vi "PC_SVG DAQ1 to TDVM DAQ2 RSS.vi"() -> ()   [LabVIEW 2021]
uses:
  Synchronization/Typedefs/Routing Path.ctl
  Synchronization/Typedefs/Routing Signal.ctl
  Signal Voltage Generation/Typedefs/Signal Generation Settings.ctl
  Signal Voltage Generation/Typedefs/Generation Types.ctl
  Signal Voltage Generation/Typedefs/Single Tone Settings.ctl
  Signal Voltage Generation/Typedefs/Waveform Type.ctl
  Signal Voltage Generation/Typedefs/Tone Settings.ctl
  Time Domain Measurement/Typedefs/Time Domain Measurements.ctl
  Time Domain Measurement/Typedefs/Timing & Trigger Settings.ctl
  Time Domain Measurement/Typedefs/Timing Settings.ctl
  Time Domain Measurement/Typedefs/Trigger Settings.ctl
  Time Domain Measurement/Typedefs/Execution Settings.ctl
  Common/Typedefs/Execution Options - Measure.ctl
  Time Domain Measurement/Typedefs/Range and Terminal Settings.ctl
  Time Domain Measurement/Typedefs/Specific Channel Settings.ctl
  Time Domain Measurement/DAQ_Time Domain Measurement.lvlib
  Synchronization/DAQ_Synchronization.lvlib
  Signal Voltage Generation/DAQ_Signal Voltage Generation.lvlib
panel:
  in  "Timing and Trigger Settings":T1={"Timing Settings"={"Sample Clock Source"="/Dev2/PFI1", "Sample Rate(Hz)"=100000.0, "Number of Samples"=10000, "Sample Timing Engine"=enum."Auto"}, "Trigger Settings"={"Trigger Type"=enum."Digital Start", "Digital Start Trigger Source"="/Dev2/PFI0", "Digital Start Trigger Edge"=10280}} {"Trigger Settings"."Digital Start Trigger Edge" items=["Rising"=10280, "Falling"=10171]; "Timing Settings"."Sample Rate(Hz)" format="%.2p"}
  out "error out":errorcluster
  out "Time Domain Measurements":T4={"Mean DC Voltage (V)"=[1.0316878948057864], "Vpp Amplitude(V)"=[2.0060539436845626], "Voltage Frequency(Hz)"=[99.99092141563642], "Voltage Waveform Period (s)"=[0.010000907940864535], "Voltage Waveform duty cycle (%)"=[50.015292519648845]} {"Voltage Waveform duty cycle (%)" format="%.2p"; "Voltage Waveform Period (s)" format="%.2p"; "Voltage Frequency(Hz)" format="%.2p"; "Vpp Amplitude(V)" format="%.2p"; "Mean DC Voltage (V)" format="%.2p"}
  out "Voltage Waveforms":waveform(dbl)[](graph)=[{"t0"=timestamp(3805341613.277684 s since 1904-01-01), "dt"=9.999999999999972e-06, "Y"=array[10000 elements], "attributes"=variant("NI_ChannelName"=variant(string "Dev2/ai0"), "NI_UnitDescription"=variant(string "Volts"))}]
  out "Generated Voltage Waveforms":waveform(dbl)[](graph)=[{"t0"=timestamp(0 s since 1904-01-01), "dt"=1e-05, "Y"=array[10000 elements]}]
  in  "Signal Generation Settings":T5={"Generation Type"=enum."Single Tone", "Generation Time (s)"=0.1, "Voltage Offset (v)"=1.0, "Single Tone Settings"={"Waveform Type"=enum."Sine Wave", "Frequency (Hz)"=100.0, "Amplitude (V)"=1.0, "Duty Cycle (%)"=50.0}, "Multi Tone Settings"=[]} {"Voltage Offset (v)" format="%.2p"; "Generation Time (s)" format="%.2p"; "Multi Tone Settings"."Amplitude (V)" format="%#.2p"; "Multi Tone Settings"."Frequency (Hz)" format="%#.2p"; "Single Tone Settings"."Duty Cycle (%)" format="%#.2p"; "Single Tone Settings"."Amplitude (V)" format="%#.2p"; "Single Tone Settings"."Frequency (Hz)" format="%#.2p"}
  in  "Routing paths":T10[](array[typedef])=[{"Signal"=enum."Start Trigger", "Output Terminal"="/Dev1/PFI0"}, {"Signal"=enum."Sample Clock", "Output Terminal"="/Dev1/PFI1"}]
  # "Frequency (Hz)"
  # "Amplitude (V)"
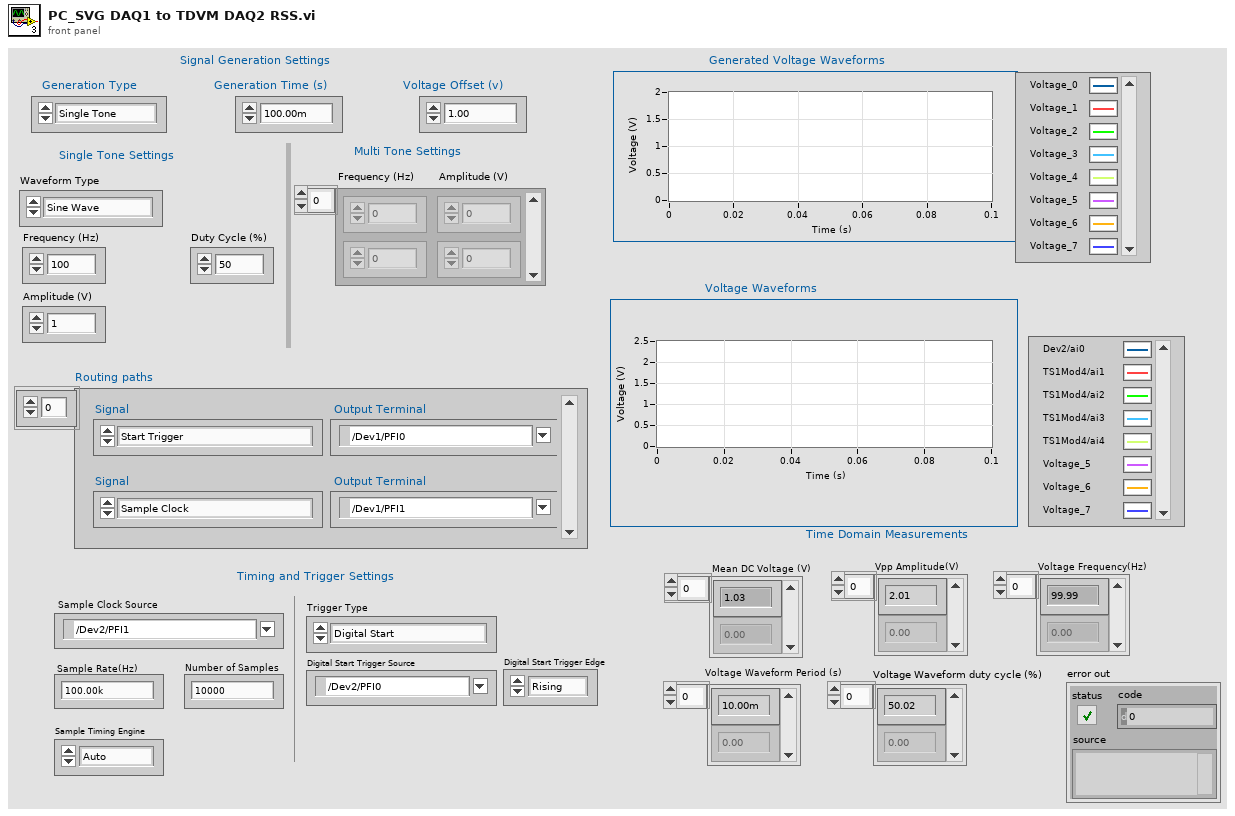
[diagram p1: front panel]
types:
  T1 = typedef "DAQ_Time Domain Measurement.lvlib/Timing & Trigger Settings.ctl" = cluster{"Timing Settings":T2, "Trigger Settings":T3}
  T2 = typedef "DAQ_Time Domain Measurement.lvlib/Timing Settings.ctl" = cluster{"Sample Clock Source":tag, "Sample Rate(Hz)":dbl, "Number of Samples":i32, "Sample Timing Engine":enum16{"te0", "te1", "ai", "Auto"}}
  T3 = typedef "DAQ_Time Domain Measurement.lvlib/Trigger Settings.ctl" = cluster{"Trigger Type":enum16{"No Trigger", "Digital Start"}, "Digital Start Trigger Source":tag, "Digital Start Trigger Edge":i32}
  T4 = typedef "DAQ_Time Domain Measurement.lvlib/Time Domain Measurements.ctl" = cluster{"Mean DC Voltage (V)":dbl[], "Vpp Amplitude(V)":dbl[], "Voltage Frequency(Hz)":dbl[], "Voltage Waveform Period (s)":dbl[], "Voltage Waveform duty cycle (%)":dbl[]}
  T5 = typedef "DAQ_Signal Voltage Generation.lvlib/Signal Generation Settings.ctl" = cluster{"Generation Type":T6, "Generation Time (s)":dbl, "Voltage Offset (v)":dbl, "Single Tone Settings":T7, "Multi Tone Settings":T9[]}
  T6 = typedef "DAQ_Signal Voltage Generation.lvlib/Generation Types.ctl" = enum16{"Single Tone", "Multi Tone"}
  T7 = typedef "DAQ_Signal Voltage Generation.lvlib/Single Tone Settings.ctl" = cluster{"Waveform Type":T8, "Frequency (Hz)":dbl, "Amplitude (V)":dbl, "Duty Cycle (%)":dbl}
  T8 = typedef "DAQ_Signal Voltage Generation.lvlib/Waveform Type.ctl" = enum16{"Sine Wave", "Square Wave"}
  T9 = typedef "DAQ_Signal Voltage Generation.lvlib/Tone Settings.ctl" = cluster{"Frequency (Hz)":dbl, "Amplitude (V)":dbl}
  T10 = typedef "DAQ_Synchronization.lvlib/Routing Path.ctl" = cluster{"Signal":T11, "Output Terminal":tag}
  T11 = typedef "DAQ_Synchronization.lvlib/Routing Signal.ctl" = enum16{"Sample Clock", "Start Trigger"}
  T12 = typedef "DAQ_Time Domain Measurement.lvlib/Range and Terminal Settings.ctl" = cluster{"Global Settings":cluster{"Min Range(V)":dbl, "Max Range(V)":dbl, "Terminal Configuration":i32}, "Specific Channel Settings":T13[]}
  T13 = typedef "DAQ_Time Domain Measurement.lvlib/Specific Channel Settings.ctl" = cluster{"Active Channels":tag, "Min Range":dbl, "Max Range":dbl, "Terminal Configuration":i32}
  T14 = typedef "DAQ_Time Domain Measurement.lvlib/Execution Settings.ctl" = cluster{"Execution option":T15, "Skip Analysis?":bool}
  T15 = typedef "Execution Options - Measure.ctl" = enum16{"Configure & Measure", "Configure only", "Measure only"}
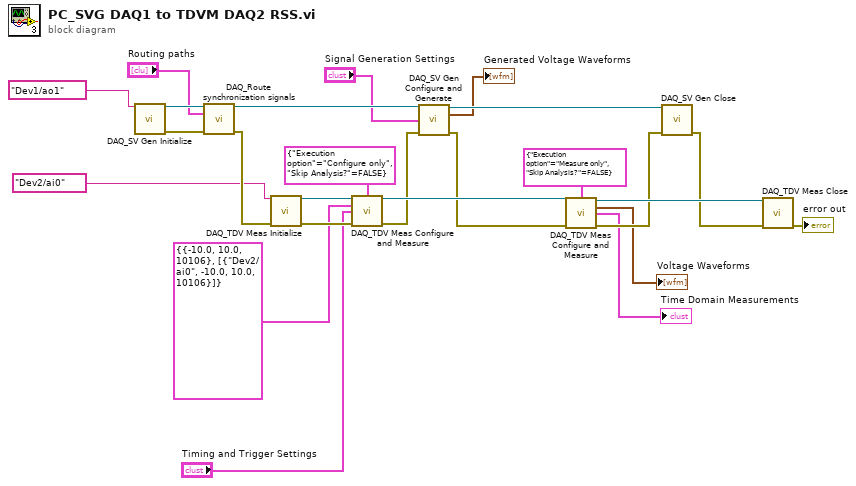
[diagram p0: block diagram]
diagram:
  n1 = call "DAQ_SV Gen Initialize.vi"("Physical Channels"=tag "Dev1/ao1") -> ("DAQmx Task Out"=w25:refnum<k21>, "error out"=w24:errorcluster)  [unwired: 13 in]
  n2 = call "DAQ_Route synchronization signals.vi"("DAQmx Task In"=w25, "Routing paths"="Routing paths", "error in"=w24) -> ("DAQmx Task Out"=w22:refnum<k21>, "error out"=w20:errorcluster)  [unwired: 11 in]
  n3 = call "DAQ_TDV Meas Initialize.vi"("Physical Channels"=tag "Dev2/ai0", "error in"=w20) -> ("DAQmx Task Out"=w19:refnum<k21>, "error out"=w16:errorcluster)  [unwired: 12 in]
  n4 = call "DAQ_TDV Meas Configure and Measure.vi"("DAQmx Task In"=w19, "Execution Settings"=T14 {"Execution option"=enum."Configure only", "Skip Analysis?"=FALSE}, "Range and Terminal Settings"=T12 {"Global Settings"={"Min Range(V)"=-10.0, "Max Range(V)"=10.0, "Terminal Configuration"=10106}, "Specific Channel Settings"=[{"Active Channels"="Dev2/ai0", "Min Range"=-10.0, "Max Range"=10.0, "Terminal Configuration"=10106}]}, "Timing and Trigger Settings"="Timing and Trigger Settings", "error in"=w16) -> ("DAQmx Task Out"=w18:refnum<k21>, "error out"=w15:errorcluster)  [unwired: 6 in, 3 out]
  n5 = call "DAQ_SV Gen Configure and Generate.vi"("DAQmx Task In"=w22, "Signal Generation Settings"="Signal Generation Settings", "error in"=w15) -> ("DAQmx Task Out"=w21:refnum<k21>, "Generated Voltage Waveforms"=→"Generated Voltage Waveforms":waveform(dbl)[], "error out"=w14:errorcluster)  [unwired: 10 in]
  n6 = call "DAQ_TDV Meas Configure and Measure.vi"("DAQmx Task In"=w18, "Execution Settings"=T14 {"Execution option"=enum."Measure only", "Skip Analysis?"=FALSE}, "error in"=w14) -> ("DAQmx Task Out"=w17:refnum<k21>, "Voltage Waveforms"=→"Voltage Waveforms":waveform(dbl)[], "Time Domain Measurements"=→"Time Domain Measurements":T4, "error out"=w11:errorcluster)  [unwired: 8 in, 1 out]
  n7 = call "DAQ_SV Gen Close.vi"("DAQmx Task In"=w21, "error in"=w11) -> ("error out"=w10:errorcluster)  [unwired: 13 in]
  n8 = call "DAQ_TDV Meas Close.vi"("DAQmx Task In"=w17, "error in"=w10) -> ("error out"=→"error out":errorcluster)  [unwired: 13 in]
